vi "FPGA Server.vi"() -> ()   [LabVIEW 2013]
doc: "This is the FPGA server for the sbRIO for the open-path cavity ring down."
uses:
  Rate.ctl
  <vilib>/Platform/TimedLoop/XDataNode/timing_clust.ctl
  <vilib>/Platform/TimedLoop/XDataNode/nitl_modes.ctl
  <vilib>/Platform/TimedLoop/XDataNode/wakeup.ctl
  <vilib>/rvi/FXPMathLib/basic elements/FxpIntAccumulator/subVIs/nifxpmath_IntAccumulator_SimConfig.ctl
  <vilib>/rvi/FXPMathLib/FxpDiv/subVIs/nifxpmath_Div_SimConfig.ctl
  <vilib>/rvi/Emulation/niFpgaSctlEmulationGetInTimedLoop.vi
  <vilib>/rvi/Emulation/niFpgaEmulationReportErrorSimple.vi
  <vilib>/rvi/Emulation/niFpgaGetClockAttributes.vi
  <vilib>/rvi/Emulation/niFpgaCriticalErrorInLSC.vi
  <vilib>/rvi/eio/common/nirviEmuTemplateMethod_errors.vi
  <vilib>/rvi/Memory/Memory_Emulation/nirvimemoryFastEmulationFpgaImpl.vi
  <instcachedir>/0/nirvimemoryFastEmulationFpgaImpl_5FBAB50466BC4C939F684F8805638BFC.lvgen/nirvimemoryFastEmulationFpgaImpl_5FBAB50466BC4C939F684F8805638BFC_003.vi
  <vilib>/rvi/DataTransferAndStorage/Container/Common/niFpgaContainerGetUniqueNameForEmu.vi
  <vilib>/rvi/Memory/Memory_Emulation/nirvimemoryFastEmulation.vi
  <vilib>/rvi/Memory/Memory_Emulation/nirvimemoryEmulation.vi
  <vilib>/rvi/interface/RandomDataEmulation/nirviRandomDataFPGAFIFO.vi
  <vilib>/rvi/interface/RandomDataEmulation/niFpgaRandomDataHandleErrors.vi
  <vilib>/rvi/Analysis/common/codeGenErrors/XNode/niFpgaXNodeCodeGenErrorHandle.vi
  <vilib>/rvi/FXPMathLib/basic elements/FxpIntAccumulator/simVIs/DllFxpIntAccumulator_sub.vi
  <vilib>/rvi/FXPMathLib/FxpDiv/simVIs/DllFxpDivTemp_sub.vi
  <vilib>/rvi/Emulation/niFpgaProcessEmulError.vi
  <vilib>/Platform/TimedLoop/XDataNode/XDataNode.xnode
  <vilib>/eio/EIONode/EIONode.xnode
  <vilib>/rvi/FXPMathLib/FxpMul/XNode/nifxpmath_Multiplier.xnode
  <vilib>/rvi/DataTransferAndStorage/Container/XNode/niFpgaContainer.xnode
  <vilib>/rvi/interface/RandomDataEmulation/nirviRandomDataFpgaReadWriteTemplate.vi
  <vilib>/rvi/Analysis/measure/mean-var-std/XNode/niFpgaMean-Var-Std.xnode
  <vilib>/rvi/FXPMathLib/basic elements/FxpIntAccumulator/XNode/nifxpmath_IntAccumulator.xnode
  <vilib>/rvi/FXPMathLib/FxpDiv/XNode/nifxpmath_Div.xnode
  <vilib>/rvi/FXPMathLib/FxpSub/XNode/nifxpmath_Sub.xnode
  <vilib>/Platform/TimedLoop/XDataNode/XDNodeRunTimeDep.lvlib
  <vilib>/rvi/FXPMathLib/sim/FxpSim.dll
panel:
  out "LF Data":T1
  in  "Low":u32 caption="Count(uSec)"
  in  "High":u32 caption="Count(uSec)"
  out "CollectData":bool
  out "Delay Ticks":u32
  in  "Delay (us)":u16
  out "RequestLaser":bool
  out "Sample Ticks":u32
  in  "Pause Digitizer":bool
  in  "Sample Time (us)":u16
  in  "Rate":T2=3 items=["1 MHz"=20, "2 MHz"=10, "2.5 MHz"=8, "5 MHz"=4, "10 MHz"=2, "20MHz"=1]
  out "LaserOFF?":bool
  in  "Cylce (ticks)":u32=40000
  out "DataRead":bool
  out "dataready":bool
  out "NewData":u16
  out "NumElements":u32
  out "Samps":u64
  in  "Stop":bool
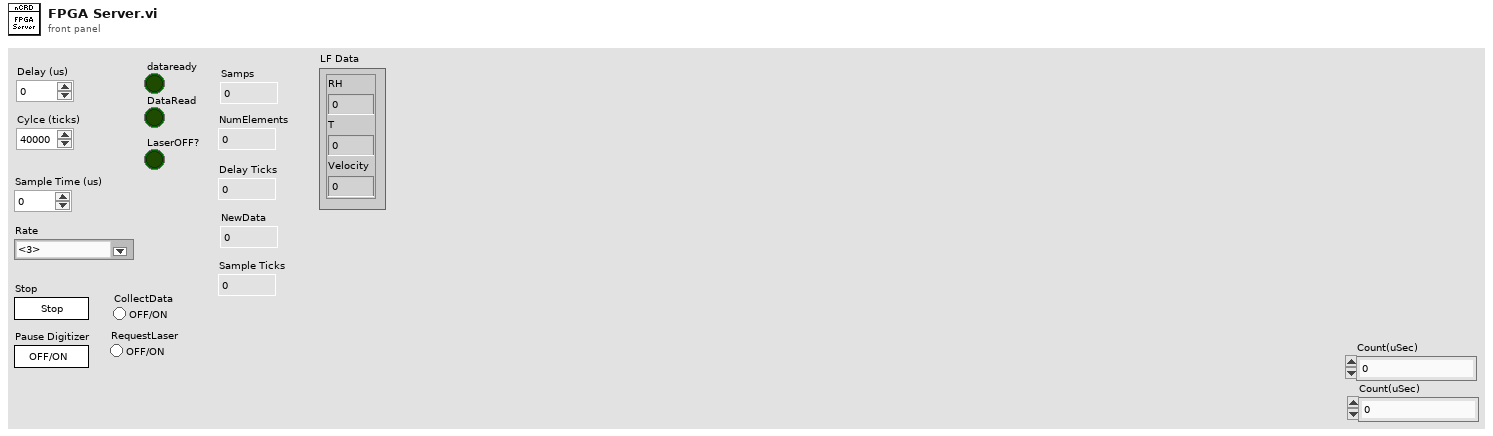
[diagram p1: front panel]
types:
  T1 = cluster{"RH":fxp<+,16,8>, "T":fxp<+/-,16,8>, "Velocity":fxp<+/-,16,8>}
  T2 = typedef "Rate.ctl" = u8
  T3 = typedef "XDNodeRunTimeDep.lvlib/timing_clust.ctl" = cluster{"Expected End [f-1]":u64, "Actual End [f-1]":u64, "Finished Late? [f-1]":bool, "Expected End [i-1]":u64, "Actual End [i-1]":u64, "Finished Late? [i-1]":bool, "Expected Start [i]":u64, "Actual Start [i]":u64, "Expected Start [f]":u64, "Actual Start [f]":u64, "Source Name":string, "Structure Name":string, "Period":i64, "Deadline":i64, "Offset":i64, "Start":i64, "Priority":i32, "Timeout":i32, "Mode":T4, "Wakeup Reason":T5, "Error":errorcluster, "Source Type":string, "Secondary Source Type":string, "Global End Time":u64, "Global Start Time":u64, "Frame Duration":u64, "Iteration Duration":u64, "Assigned CPU":i32, "I/O Scan Engine Mode":u32}
  T4 = typedef "XDNodeRunTimeDep.lvlib/nitl_modes.ctl" = enum32{"No Change", "Process missed periods, maintain original phase", "Discard missed periods, maintain original phase", "Process missed periods, ignore original phase", "Discard missed periods, ignore original phase"}
  T5 = typedef "XDNodeRunTimeDep.lvlib/wakeup.ctl" = enum32{"Normal", "Aborted", "Asynchronous wakeup", "Timing source error", "Timed loop error", "Timeout"}
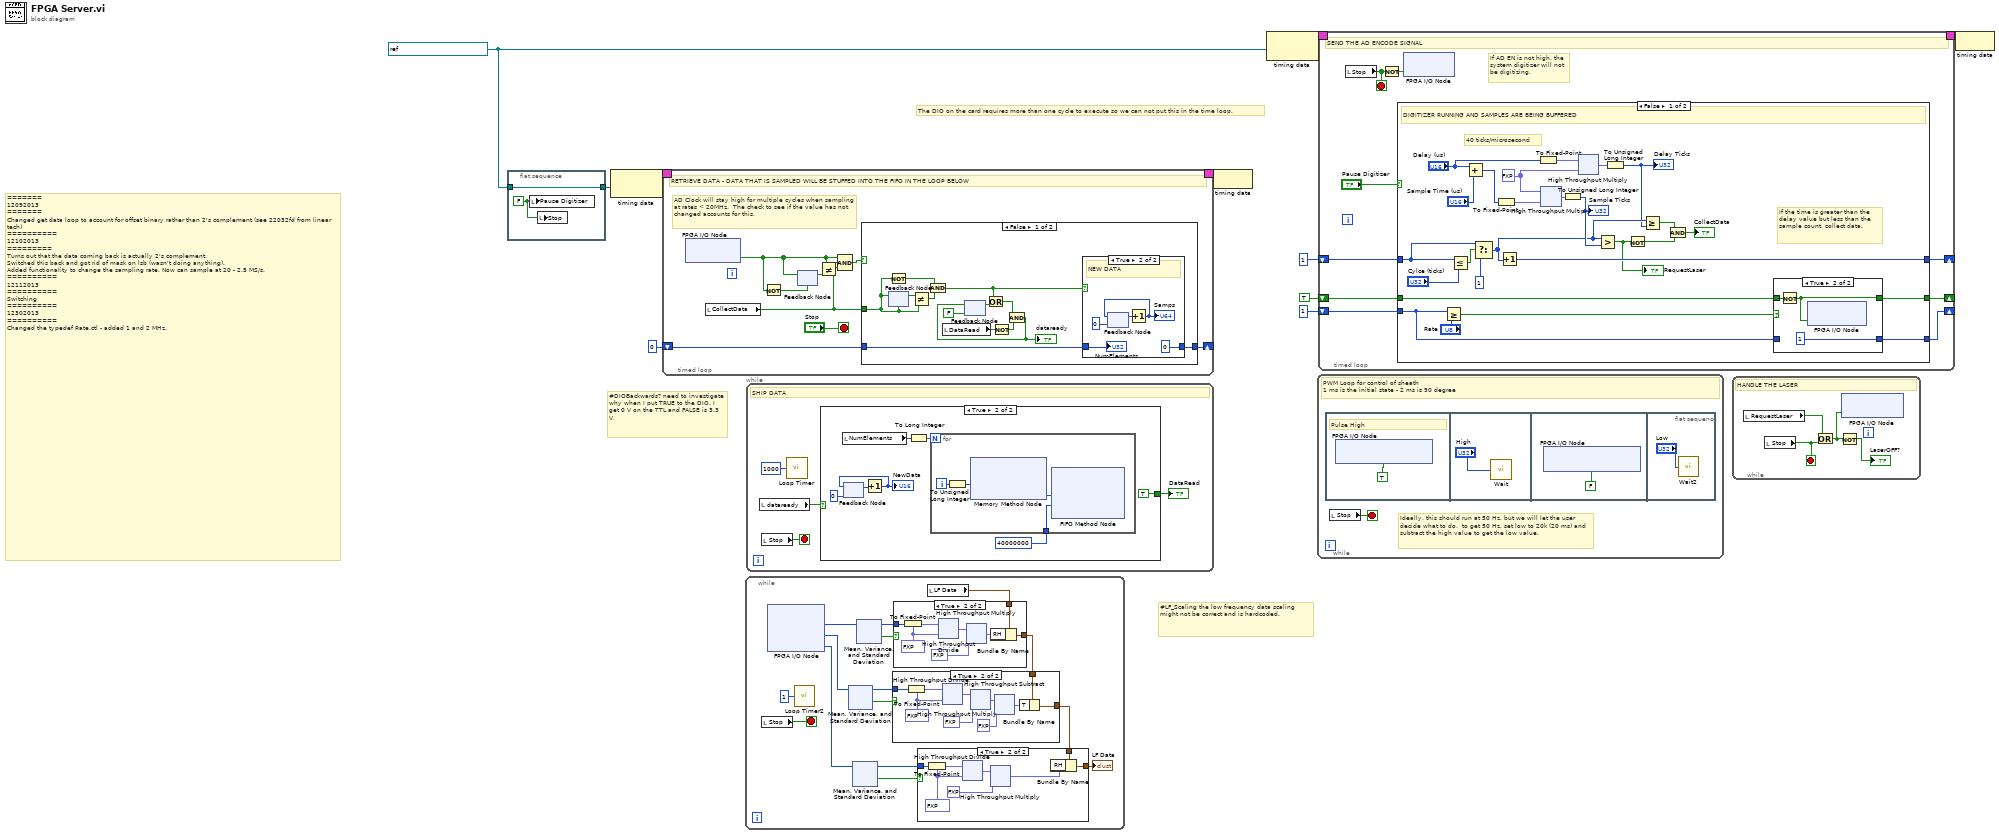
[diagram p0: block diagram]
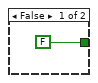
[diagram p5: hidden frame]
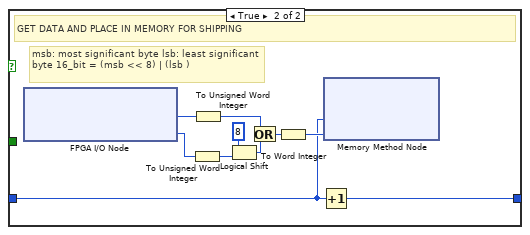
[diagram p7: hidden frame]
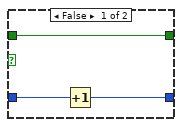
[diagram p8: hidden frame]
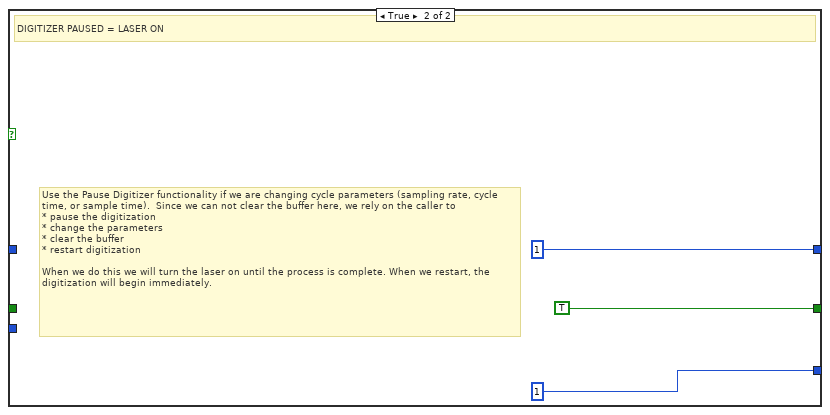
[diagram p9: hidden frame]
diagram:
  w2 = refnum<k21> "40 MHz Onboard Clock" ("Source Name")
  # "#LF_Scaling the low frequency data scaling might not be correct and is hardcoded."
  # "The DIO on the card requires more than one cycle to execute so we can not put this in the time loop."
  # "#DIOBackwards? need to investigate why when I put TRUE to the DIO, I get 0 V on the TTL and FALSE is 3.3 V."
  # "=======\n12092013 \n=======\nChanged get data loop to account for offset binary rather than 2's complement (see 22032fd from linear tech)\n==========\n12102013\n=========\nTurns out that the data coming back is actually 2's complement. \nSwitched this back and got rid of mask on lsb (wasn't doing anything).\nAdded functionality to change the sampling rate. Now can sample at 20 - 2.5 MS/s.\n==========\n12112013\n==========\nSwitching\n==========\n12302013\n==========\nChanged the typedef Rate.ctl - added 1 and 2 MHz."
  n1 = flat-sequence {
    tunnel: w2 -> [w12]
    tunnel: [w12] -> w1
    frame #0 {
      w11 = FALSE ("Pause Digitizer")
      n2 = local write "Pause Digitizer"(w11) -> ()
      n3 = local write "Stop"(w11) -> ()
    }
  }
  n4 = node-c288(w1) -> (w8:T3)
  n5 = timed-loop {
    timing: w8 -> [_]
    timing-out: [_] -> w7
    shift-right: [w19] -> _
    shift-left: u32 0 -> [w20]
    stop <- "Stop" stop-if-true
    # "AD Clock will stay high for multiple cycles when sampling at rates < 20MHz.  The check to see if the value has not changed accounts for this."
    # "RETRIEVE DATA - DATA THAT IS SAMPLED WILL BE STUFFED INTO THE FIFO IN THE LOOP BELOW"
    n6 = xnode "FPGA I/O Node"() -> ("AD CLK"=w18:bool)  [unwired: 1 in, 1 out]
    n7 = local read "CollectData"() -> (w13:bool)
    n8 = Not(x=w18) -> (.not. x?=w17:bool)
    n9 = feedback-in #1(w18) -> ()
    n10 = feedback #1(w17) -> (w16:bool)
    n11 = Not Equal?(x=w18, y=w16) -> (x != y?=w15:bool)
    n12 = Compound Arithmetic op=AND(w18, w15, w13) -> (w14:bool)
    n13 = case shown="False" w14 {
      tunnel: w13 -> [w33 _]
      tunnel: w20 -> [w30 w43]
      tunnel: [w29 w42] -> w19
      frame False {
        n14 = Not(x=w33) -> (.not. x?=w31:bool)
        n15 = feedback-in #2(w33) -> ()
        n16 = feedback #2(w33) -> (w34:bool)
        n17 = Not Equal?(x=w34, y=w33) -> (x != y?=w32:bool)
        n18 = And(x=w31, y=w32) -> (x .and. y?=w25:bool)
        n19 = local read "DataRead"() -> (w26:bool)
        n20 = feedback #3(FALSE) -> (w24:bool)
        n21 = Or(x=w25, y=w24) -> (x .or. y?=w23:bool)
        n22 = Not(x=w26) -> (.not. x?=w27:bool)
        n23 = And(x=w23, y=w27) -> (x .and. y?=w22:bool)
        "dataready" <- w22
        n24 = feedback-in #3(w22) -> ()
        n25 = case shown="True" w25 {
          tunnel: w30 -> [w35 w36]
          tunnel: [w35 u32 0] -> w29
          frame False {
          }
          frame True {
            # "NEW DATA"
            n26 = feedback #4(u64 0) -> (w39:u64)
            n27 = Increment(x=w39) -> (x+1=w38:u64)
            "Samps" <- w38
            n28 = feedback-in #4(w38) -> ()
            "NumElements" <- w36
          }
        }
      }
      frame True {
        # "msb: most significant byte lsb: least significant byte 16_bit = (msb << 8) | (lsb )"
        # "GET DATA AND PLACE IN MEMORY FOR SHIPPING"
        n29 = xnode "FPGA I/O Node"() -> ("RMC/LVTTL/DIO7:0"=w50:u8, "RMC/LVTTL/DIO15:8"=w41:u8)  [unwired: 2 in, 2 out]
        n30 = To Unsigned Word Integer(number=w41) -> (unsigned 16bit integer=w46:u16)
        n31 = To Unsigned Word Integer(number=w50) -> (unsigned 16bit integer=w48:u16)
        n32 = Logical Shift(y=i16 8, x=w46) -> (x << y=w47:u16)
        n33 = Or(x=w48, y=w47) -> (x .or. y?=w45:u16)
        n34 = To Word Integer(number=w45) -> (16bit integer=w44:i16)
        n35 = Increment(x=w43) -> (x+1=w42:u32)
        n36 = xnode ("Memory Method Node")("Address"=w43, "Data"=w44) -> ()  [unwired: 1 in, 1 out]
      }
    }
  }
  n37 = while {
    stop <- w53 stop-if-true
    n38 = local read "Stop"() -> (w53:bool)
    n39 = xnode "FPGA I/O Node"() -> ("RH"=w66:i16, "T"=w65:i16, "Velocity"=w58:i16)  [unwired: 3 in, 3 out]
    n40 = call "Loop Timer2"("Count(mSec)"=u32 1 ("Count(Ticks)")) -> ()  [unwired: 1 out]
    n41 = xnode "Mean, Variance, and Standard Deviation"("input data"=w65) -> ("mean"=w60:i16, "output valid"=w61:bool)  [unwired: 1 in]
    n42 = xnode "Mean, Variance, and Standard Deviation"("input data"=w58) -> ("mean"=w56:i16, "output valid"=w57:bool)  [unwired: 1 in]
    n43 = xnode "Mean, Variance, and Standard Deviation"("input data"=w66) -> ("mean"=w63:i16, "output valid"=w62:bool)  [unwired: 1 in]
    n44 = local read "LF Data"() -> (w64:T1)
    n45 = case shown="True" w62 {
      tunnel: w64 -> [w214 w222]
      tunnel: w63 -> [_ w221]
      tunnel: [w214 w215] -> w59
      frame False {
      }
      frame True {
        w219 = fxp<+/-,16,16> 32767.0
        n46 = To Fixed-Point(fixed-point type=w219, number=w221) -> (fixed-point=w220:fxp<+/-,16,16>)
        n47 = xnode "High Throughput Divide"("x"=w220, "y"=w219) -> ("x/y"=w218:fxp<+/-,16,1>)
        n48 = xnode "High Throughput Multiply"("x"=w218, "y"=fxp<+,8,8> 200.0) -> ("x*y"=w216:fxp<+/-,24,9>)
        n49 = Bundle By Name(cluster=w222, "RH"=w216) -> (w215:T1)
      }
    }
    n50 = case shown="True" w61 {
      tunnel: w59 -> [w176 w186]
      tunnel: w60 -> [_ w185]
      tunnel: [w176 w177] -> w55
      frame False {
      }
      frame True {
        w183 = fxp<+/-,16,16> 32767.0
        n51 = To Fixed-Point(fixed-point type=w183, number=w185) -> (fixed-point=w184:fxp<+/-,16,16>)
        n52 = xnode "High Throughput Divide"("x"=w184, "y"=w183) -> ("x/y"=w182:fxp<+/-,16,1>)
        n53 = xnode "High Throughput Multiply"("x"=w182, "y"=fxp<+,8,8> 240.0) -> ("x*y"=w180:fxp<+/-,24,9>)
        n54 = xnode "High Throughput Subtract"("x"=w180, "y"=fxp<+/-,8,8> 40.0) -> ("x-y"=w178:fxp<+/-,25,10>)
        n55 = Bundle By Name(cluster=w186, "T"=w178) -> (w177:T1)
      }
    }
    n56 = case shown="True" w57 {
      tunnel: w55 -> [w140 w148]
      tunnel: w56 -> [_ w147]
      tunnel: [w140 w141] -> w54
      frame False {
      }
      frame True {
        w145 = fxp<+/-,16,16> 32767.0
        n57 = To Fixed-Point(fixed-point type=w145, number=w147) -> (fixed-point=w146:fxp<+/-,16,16>)
        n58 = xnode "High Throughput Divide"("x"=w146, "y"=w145) -> ("x/y"=w144:fxp<+/-,16,1>)
        n59 = xnode "High Throughput Multiply"("x"=w144, "y"=fxp<+,8,8> 10.0) -> ("x*y"=w142:fxp<+/-,24,9>)
        n60 = Bundle By Name(cluster=w148, "RH"=w142) -> (w141:T1)
      }
    }
    "LF Data" <- w54
  }
  n61 = while {
    stop <- w397 stop-if-true
    # "SHIP DATA"
    n62 = local read "dataready"() -> (w396:bool)
    n63 = local read "Stop"() -> (w397:bool)
    n64 = call "Loop Timer"("Count(Ticks)"=u32 1000) -> ()  [unwired: 1 out]
    n65 = case shown="True" w396 {
      tunnel: [FALSE TRUE] -> w395
      frame False {
      }
      frame True {
        n66 = local read "NumElements"() -> (w399:u32)
        n67 = feedback #5(u16 0) -> (w403:u16)
        n68 = Increment(x=w403) -> (x+1=w404:u16)
        "NewData" <- w404
        n69 = feedback-in #5(w404) -> ()
        n70 = To Long Integer(number=w399) -> (32bit integer=w400:i32)
        n71 = for {
          N: w400 -> [_]
          tunnel: 40000000 ("Timeout") -> [w409]
          i -> [w408]
          n72 = To Unsigned Long Integer(number=w408) -> (unsigned 32bit integer=w406:u32)
          n73 = xnode ("Memory Method Node")("Address"=w406) -> ("Data"=w407:i16)  [unwired: 1 in, 1 out]
          n74 = xnode ("FIFO Method Node")("Element"=w407, "Timeout"=w409) -> ()  [unwired: 1 in, 2 out]
        }
      }
    }
    "DataRead" <- w395
  }
  n75 = node-c288(w7) -> ()
  n76 = node-c288(w2) -> (w10:T3)
  n77 = while {
    stop <- w410 stop-if-true
    # "Ideally, this should run at 50 Hz, but we will let the user decide what to do.  to get 50 Hz, set low to 20k (20 ms) and subtract the high value to get the low value."
    # "PWM Loop for control of sheath\n1 ms is the initial state - 2 ms is 90 degree"
    n78 = flat-sequence {
      frame #0 {
        # "Pulse High"
        n79 = xnode "FPGA I/O Node"("RMC/Sinking/DO14"=TRUE ("Mod4/DIO0")) -> ()  [unwired: 1 in, 1 out]
      }
      frame #1 {
        n80 = call "Wait"("Count(uSec)"="High") -> ()  [unwired: 1 out]
      }
      frame #2 {
        n81 = xnode "FPGA I/O Node"("RMC/Sinking/DO14"=FALSE ("Mod4/DIO0")) -> ()  [unwired: 1 in, 1 out]
      }
      frame #3 {
        n82 = call "Wait2"("Count(uSec)"="Low") -> ()  [unwired: 1 out]
      }
    }
    n83 = local read "Stop"() -> (w410:bool)
  }
  n84 = timed-loop {
    shift-right: [w418] -> _
    shift-left: TRUE -> [w419]
    timing: w10 -> [_]
    timing-out: [_] -> w9
    shift-right: [w420] -> _
    shift-left: u32 1 -> [w421]
    shift-right: [w417] -> _
    shift-left: u8 1 -> [w416]
    stop <- w422 stop-if-true
    # "If AD EN is not high, the system digitizer will not be digitizing."
    # "SEND THE AD ENCODE SIGNAL"
    n85 = local read "Stop"() -> (w422:bool)
    n86 = Not(x=w422) -> (.not. x?=w423:bool)
    n87 = case shown="False" "Pause Digitizer" {
      tunnel: w421 -> [w446 _]
      tunnel: [w445 u32 1] -> w420
      tunnel: w419 -> [w442 _]
      tunnel: [w441 TRUE ("Element")] -> w418
      tunnel: [w440 u8 1] -> w417
      tunnel: w416 -> [w439 _]
      frame False {
        w429 = fxp<+,8,8> 40.0 ("Sample Time (us) 2")
        # "40 ticks/microsecond"
        # "If the time is greater than the delay value but less than the sample count, collect data."
        # "DIGITIZER RUNNING AND SAMPLES ARE BEING BUFFERED"
        n88 = Greater Or Equal?(x=w439, y="Rate") -> (x >= y?=w443:bool)
        n89 = Less Or Equal?(x=w446, y="Cylce (ticks)") -> (x <= y?=w448:bool)
        n90 = Add(x="Delay (us)", y="Sample Time (us)") -> (x+y=w434:u16)
        n91 = Select(t=w446, s=w448, f=u32 1) -> (s? t:f=w427:u32)
        n92 = To Fixed-Point(number=w434) -> (fixed-point=w437:fxp<+,16,16>)  [unwired: 1 in]
        n93 = Increment(x=w427) -> (x+1=w445:u32)
        n94 = To Fixed-Point(number="Delay (us)") -> (fixed-point=w430:fxp<+,16,16>)  [unwired: 1 in]
        n95 = xnode ("High Throughput Multiply")("x"=w429, "y"=w437) -> ("x*y"=w438:fxp<+,32,32>)
        n96 = To Unsigned Long Integer(number=w438) -> (unsigned 32bit integer=w436:u32)
        "Sample Ticks" <- w436
        n97 = xnode ("High Throughput Multiply")("x"=w430, "y"=w429) -> ("x*y"=w428:fxp<+,32,32>)
        n98 = Greater?(x=w427, y=w436) -> (0:w433:bool)
        "RequestLaser" <- w433
        n99 = To Unsigned Long Integer(number=w428) -> (unsigned 32bit integer=w425:u32)
        "Delay Ticks" <- w425
        n100 = Not(x=w433) -> (.not. x?=w432:bool)
        n101 = Greater Or Equal?(x=w427, y=w425) -> (x >= y?=w426:bool)
        n102 = And(x=w426, y=w432) -> (x .and. y?=→"CollectData":bool)
        n103 = case shown="True" w443 {
          tunnel: w442 -> [w452 w455]
          tunnel: [w452 w454] -> w441
          tunnel: [w450 u8 1] -> w440
          tunnel: w439 -> [w451 _]
          frame False {
            n104 = Increment(x=w451) -> (x+1=w450:u8)
          }
          frame True {
            n105 = Not(x=w455) -> (.not. x?=w454:bool)
            n106 = xnode "FPGA I/O Node"("ENCODE"=w454) -> ()  [unwired: 1 in, 1 out]
          }
        }
      }
      frame True {
        # "Use the Pause Digitizer functionality if we are changing cycle parameters (sampling rate, cycle time, or sample time).  Since we can not clear the buffer here, we rely on the caller to \n* pause the digitization\n* change the parameters\n* clear the buffer\n* restart digitization\n\nWhen we do this we will turn the laser on until the process is complete. When we restart, the digitization will begin immediately."
        # "DIGITIZER PAUSED = LASER ON"
      }
    }
    n107 = xnode "FPGA I/O Node"("AD EN"=w423) -> ()  [unwired: 1 in, 1 out]
  }
  n108 = while {
    stop <- w463 stop-if-true
    # "HANDLE THE LASER"
    n109 = local read "RequestLaser"() -> (w464:bool)
    n110 = local read "Stop"() -> (w463:bool)
    n111 = Or(x=w464, y=w463) -> (x .or. y?=w462:bool)
    n112 = Not(x=w462) -> (.not. x?=→"LaserOFF?":bool)
    n113 = xnode "FPGA I/O Node"("Laser Out"=w462) -> ()  [unwired: 1 in, 1 out]
  }
  n114 = node-c288(w9) -> ()
